vi "svc_Get Y-Axis Strings.vi"(9 "y-axis unit label":string, 10 "y-axis units":T1 items=["Band Power"=11, "Specific Loudness"=12, "Time Varying Loudness"=13, "Specific Sharpness"=14, "Specific Roughness"=15, "Specific Fluctuation Strength"=16, "Loudness"=21, "Level"=22, "Sharpness"=23, "Roughness"=24, "Fluctuation Strength"=25]) -> (1 "y-axis unit string":string, 2 "y-axis label":string)   [LabVIEW 2017]
uses:
  <vilib>/addons/_NISVFA/_Shared subVIs/Controls/svc_Y-Axis Units.ctl
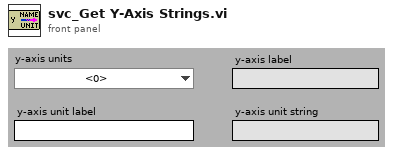
[diagram p1: front panel]
types:
  T1 = typedef "svc_Y-Axis Units.ctl" = u16
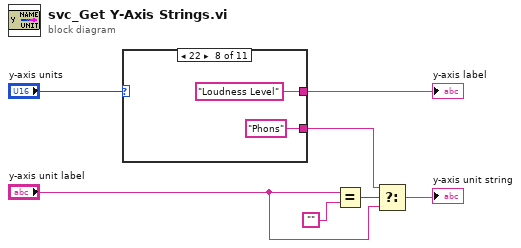
[diagram p0: block diagram]
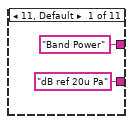
[diagram p2: hidden frame]
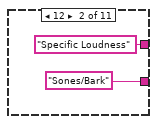
[diagram p3: hidden frame]
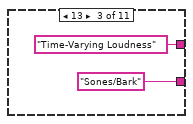
[diagram p4: hidden frame]
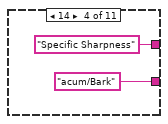
[diagram p5: hidden frame]
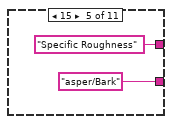
[diagram p6: hidden frame]
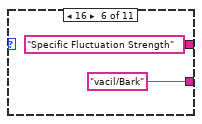
[diagram p7: hidden frame]
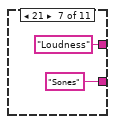
[diagram p8: hidden frame]
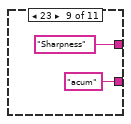
[diagram p9: hidden frame]
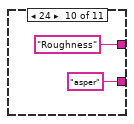
[diagram p10: hidden frame]
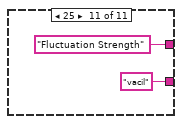
[diagram p11: hidden frame]
diagram:
  n1 = case shown="22" "y-axis units" {
    tunnel: ["Band Power" ("channel name") "Specific Loudness" ("channel name") "Time-Varying Loudness" ("channel name") "Specific Sharpness" ("channel name") "Specific Roughness" ("channel name") "Specific Fluctuation Strength" ("channel name") "Loudness" ("channel name") "Loudness Level" ("channel name") "Sharpness" ("channel name") "Roughness" ("channel name") "Fluctuation Strength" ("channel name")] -> w7
    tunnel: ["dB ref 20u Pa" "Sones/Bark" "Sones/Bark" "acum/Bark" "asper/Bark" "vacil/Bark" "Sones" "Phons" "acum" "asper" "vacil"] -> w3
    frame 11, Default {
    }
    frame 12 {
    }
    frame 13 {
    }
    frame 14 {
    }
    frame 15 {
    }
    frame 16 {
    }
    frame 21 {
    }
    frame 22 {
    }
    frame 23 {
    }
    frame 24 {
    }
    frame 25 {
    }
  }
  "y-axis label" <- w7
  n2 = Equal?(x="y-axis unit label", y="") -> (x = y?=w5:bool)
  n3 = Select(t=w3, s=w5, f="y-axis unit label") -> (s? t:f=→"y-axis unit string":string)
